vi "USB_WeatherLink_Serialnumber.vi"() -> ()   [LabVIEW 2013]
panel:
  out "WeatherLink USB serial number":u32
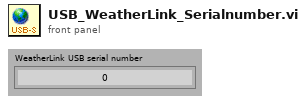
[diagram p1: front panel]
diagram:
